vi "ParseSysexCapabilityResponse.vi"(8 "error in":errorcluster={"status"=FALSE, "code"=1073676294, "source"="VISA Read in SerialCommunication.Transport.vi->TransportWrapper.vi->Capability Query.vi->Example.api.vi"}, 10 "Sysex Message":u8[](array[numeric])=[240, 108, 127, 127, 0, 1, 11, 1, 1, 1, 4, 14, 127, 0, 1, 11, 1, 1, 1, 3, 8, 4, 14, 127, 0, 1, 11, 1, 1, 1, 4, 14, 127, 0, 1, 11, 1, 1, 1, 3, 8, 4, 14, 127, 0, 1, 11, 1, 1, 1, 3, 8, 4, 14, 127, 0, 1, 11, 1, 1, 1, 4, 14, 127, 0, 1, 11, 1, 1, 1, 4, 14, 127, 0, 1, 11, 1, 1, 1, 3, 8, 4, 14, 127, 0, 1, 11, 1, 1, 1, 3, 8, 4, 14, 127, 0, 1, 11, 1, 1, 1, 3, 8, 4, 14, 127, 0, 1, 11, 1, 1, 1, 4, 14, 127, 0, 1, 11, 1, 1, 1, 4, 14, 127, 0, 1, 11, 1, 1, 1, 2, 10, 4, 14, 127, 0, 1, 11, 1, 1, 1, 2, 10, 4, 14, 127, 0, 1, 11, 1, 1, 1, 2, 10, 4, 14, 127, 0, 1, 11, 1, 1, 1, 2, 10, 4, 14, 127, 0, 1, 11, 1, 1, 1, 2, 10, 4, 14, 6, 1, 127, 0, 1, 11, 1, 1, 1, 2, 10, 4, 14, 6, 1, 127, 247] format="%x") -> (0 "error out":errorcluster={"status"=FALSE, "code"=1073676294, "source"="VISA Read in SerialCommunication.Transport.vi->TransportWrapper.vi->Capability Query.vi->Example.api.vi"}, 1 "IsValidSysex":bool=TRUE)   [LabVIEW 2020, in "FirmataClient.lvlib"]
doc: "Parse a message according to the Firmata Protocol Requirements. \n- https://github.com/firmata/protocol\n- https://github.com/firmata/protocol/blob/master/protocol.md"
uses:
  Controls/FirmataProtocolConstants.ctl
  FirmataClient.lvlib
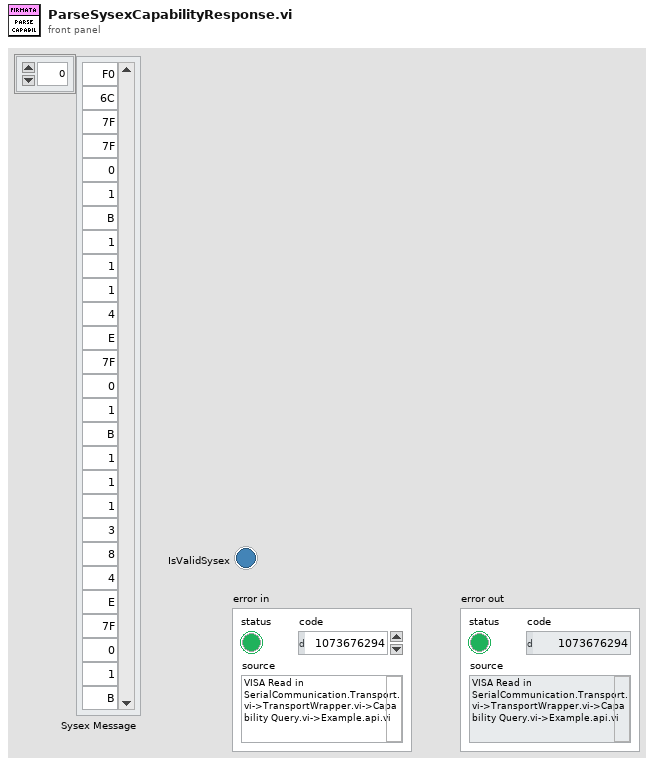
[diagram p1: front panel]
types:
  T1 = typedef "FirmataClient.lvlib/FirmataProtocolConstants.ctl" = u16
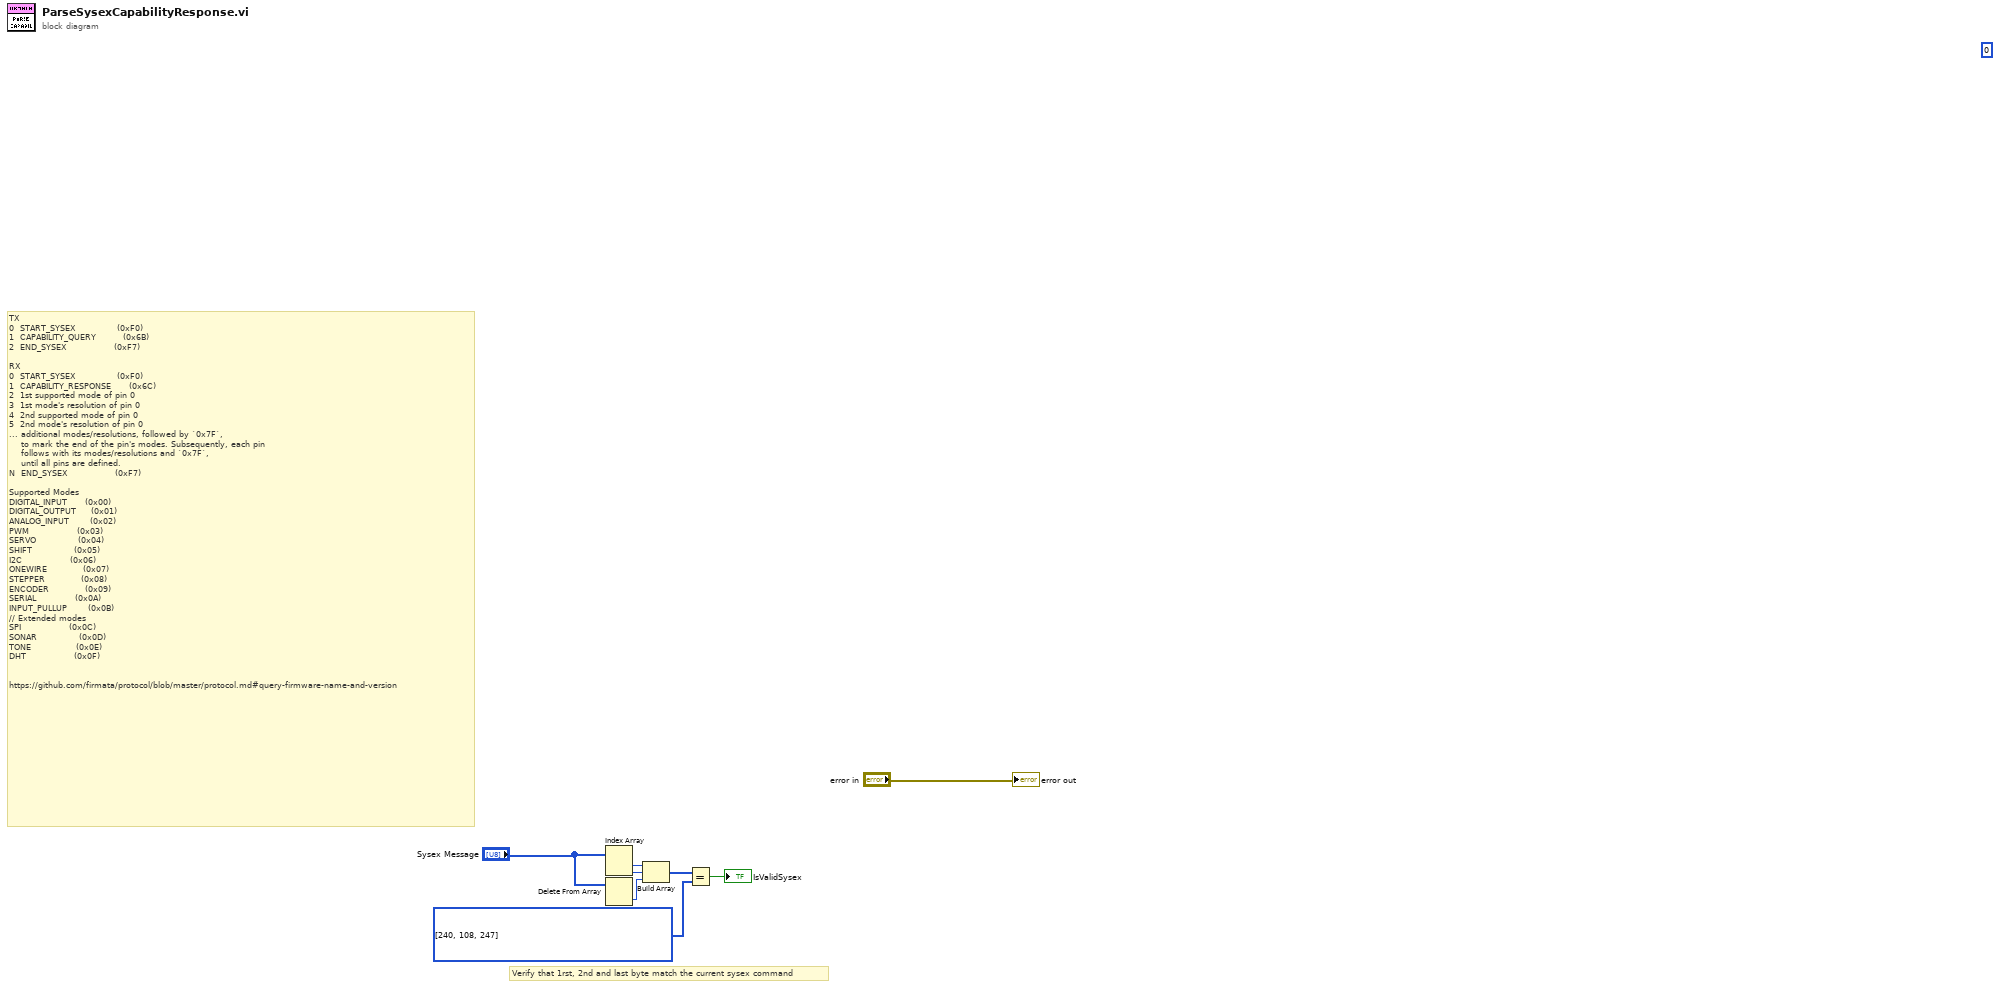
[diagram p0: block diagram]
diagram:
  (unwired) 0
  w2 = T1[] [240, 108, 247] items=["ANALOG_IO_MESSAGE"=224, "DIGITAL_IO_MESSAGE"=144, "REPORT_ANALOG_PIN"=192, "REPORT_DIGITAL_PORT"=208, "START_SYSEX"=240, "END_SYSEX"=247, "SET_PIN_MODE"=244, "SET_DIGITAL_PIN_VALUE"=245, "PROTOCOL_VERSION"=249, "SYSTEM_RESET"=255, "SYSEX.EXTENDED_ID"=0, "SYSEX.RESERVED_USER_COMMANDs"=1, "SYSEX.ANALOG_MAPPING_QUERY"=105, "SYSEX.ANALOG_MAPPING_RESPONSE"=106, "SYSEX.CAPABILITY_QUERY"=107, "SYSEX.CAPABILITY_RESPONSE"=108, "SYSEX.PIN_STATE_QUERY"=109, "SYSEX.PIN_STATE_RESPONSE"=110, "SYSEX.REPORT_FIRMWARE"=121, "SYSEX.EXTENDED_ANALOG"=111, "SYSEX.STRING_DATA"=113, "SYSEX.REALTIME"=127, "SYSEX.NON_REALTIME"=126, "SYSEX.SAMPLING_INTERVAL"=122, "FEATURES.SYSEX.I2C_READ_WRITE"=118, "FEATURES.SYSEX.I2C_REPLY"=119, "FEATURES.SYSEX.I2C_CONFIG"=120]
  # "Verify that 1rst, 2nd and last byte match the current sysex command"
  # "TX\n0  START_SYSEX              (0xF0)\n1  CAPABILITY_QUERY         (0x6B)\n2  END_SYSEX                (0xF7)\n\nRX\n0  START_SYSEX              (0xF0)\n1  CAPABILITY_RESPONSE      (0x6C)\n2  1st supported mode of pin 0\n3  1st mode's resolution of pin 0\n4  2nd supported mode of pin 0\n5  2nd mode's resolution of pin 0\n... additional modes/resolutions, followed by `0x7F`,\n    to mark the end of the pin's modes. Subsequently, each pin\n    follows with its modes/resolutions and `0x7F`,\n    until all pins are defined.\nN  END_SYSEX                (0xF7)\n\nSupported Modes\nDIGITAL_INPUT      (0x00)\nDIGITAL_OUTPUT     (0x01)\nANALOG_INPUT       (0x02)\nPWM                (0x03)\nSERVO              (0x04)\nSHIFT              (0x05)\nI2C                (0x06)\nONEWIRE            (0x07)\nSTEPPER            (0x08)\nENCODER            (0x09)\nSERIAL             (0x0A)\nINPUT_PULLUP       (0x0B)\n// Extended modes \nSPI                (0x0C)\nSONAR              (0x0D)\nTONE               (0x0E)\nDHT                (0x0F)\n\n\nhttps://github.com/firmata/protocol/blob/master/protocol.md#query-firmware-name-and-version"
  n1 = Index Array(array="Sysex Message") -> (element #1=w8:u8, element #2=w6:u8)  [unwired: 2 in]
  n2 = Delete From Array(array="Sysex Message") -> (deleted portion=w7:u8)  [unwired: 2 in, 1 out]
  n3 = Build Array(w8, w6, w7) -> (w5:u8[])
  n4 = Equal?(x=w5, y=w2) -> (x = y?=→"IsValidSysex":bool)
  "error out" <- "error in"
